vi "Update Clock.vi"(6 "timeout (ms)":i32=1000, 8 "error in":errorcluster, 10 "Clock Update":T1, 11 "gRPC ID in":T3) -> (0 "error out":errorcluster, 3 "gRPC ID out":T3)   [LabVIEW 2021, in "CIFManagerClientWrapper.lvlib"]
uses:
  CIFManagerClientWrapper.lvlib
  <vilib>/gRPC/LabVIEW gRPC Library/Shared/grpcId.ctl
  <vilib>/CIF Foundation/CIF Utilities/Time/Typedef/Clock Update.ctl
  <vilib>/CIF Foundation/CIF Utilities/Time/Typedef/Timestamp Pair.ctl
  CIF_Manager_client/RPC Messages/cif_manager_UpdateClockRequest.ctl
  CIF_Manager_client/RPC Messages/cif_manager_TimePair.ctl
  CIF_Manager_client/CIF_Manager_client.lvlib
  <vilib>/gRPC/LabVIEW gRPC Library/grpc-lvsupport-release.lvlib
  <vilib>/CIF Foundation/CIF Utilities/Time/Time_CIF_U.lvlib
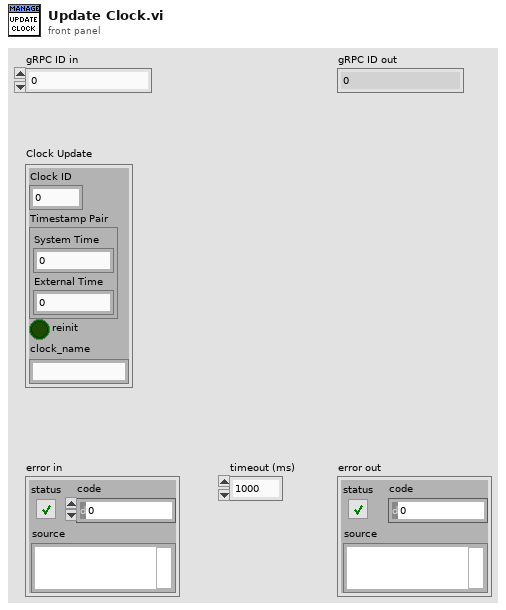
[diagram p1: front panel]
types:
  T1 = typedef "Time_CIF_U.lvlib/Clock Update.ctl" = cluster{"Clock ID":u8, "Timestamp Pair":T2, "reinit":bool, "clock_name":string}
  T2 = typedef "Time_CIF_U.lvlib/Timestamp Pair.ctl" = cluster{"System Time":i64, "External Time":i64}
  T3 = typedef "grpc-lvsupport-release.lvlib/grpcId.ctl" = u64
  T4 = typedef "CIF_Manager_client.lvlib/cif_manager_UpdateClockRequest.ctl" = cluster{"clock_id":u32, "timestamp_pair":T5, "reinit":bool, "clock_name":string}
  T5 = typedef "CIF_Manager_client.lvlib/cif_manager_TimePair.ctl" = cluster{"system_time":i64, "external_time":i64}
  T6 = typedef "CIF_Manager_client.lvlib/cif_manager_UpdateClockResponse.ctl" = cluster{"status":T7}
  T7 = typedef "CIF_Manager_client.lvlib/cif_common_Status.ctl" = cluster{"code":i32, "message":string}
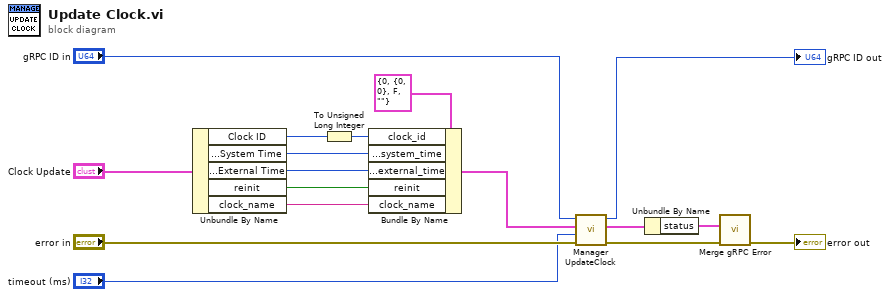
[diagram p0: block diagram]
diagram:
  n1 = Unbundle By Name("Clock Update") -> ("Clock ID"=w9:u8, "Timestamp Pair.System Time"=w5:i64, "Timestamp Pair.External Time"=w6:i64, "reinit"=w7:bool, "clock_name"=w8:string)
  n2 = To Unsigned Long Integer(number=w9) -> (unsigned 32bit integer=w4:u32)
  n3 = Bundle By Name(cluster=T4 {"clock_id"=0, "timestamp_pair"={"system_time"=0, "external_time"=0}, "reinit"=FALSE, "clock_name"=""} ("Request Data"), "clock_id"=w4, "timestamp_pair.system_time"=w5, "timestamp_pair.external_time"=w6, "reinit"=w7, "clock_name"=w8) -> (w10:T4)
  n4 = call "Manager UpdateClock.vi"("error in"="error in", "timeout (ms)"="timeout (ms)", "Request Data"=w10, "gRPC ID"="gRPC ID in") -> ("error out"=w13:errorcluster, "Response Data"=w2:T6, "gRPC ID out"=→"gRPC ID out":T3)  [unwired: 5 in]
  n5 = Unbundle By Name(w2) -> ("status"=w1:T7)
  n6 = call "Merge gRPC Error.vi"("error in (no error)"=w13, "gRPC Error"=w1) -> ("error out"=→"error out":errorcluster)  [unwired: 9 in]
